vi "sonarPY.vi"(8 "error in (no error)":errorcluster, 11 "目標":dbl) -> (0 "error out":errorcluster, 3 "公分":dbl(slide) scale=0.0..200.0)   [LabVIEW 2019]
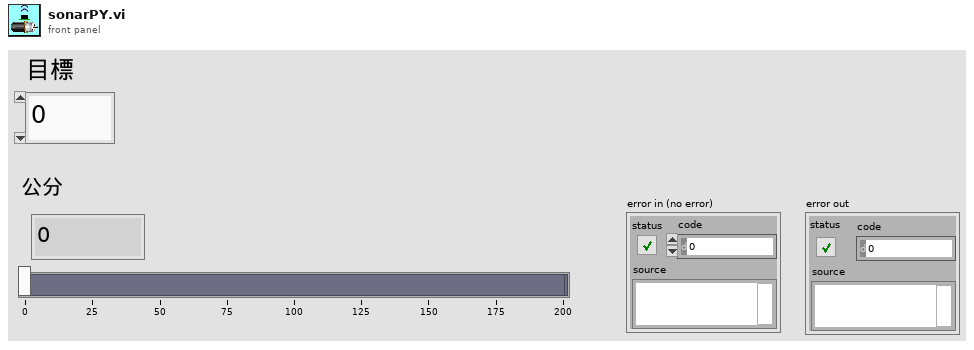
[diagram p1: front panel]
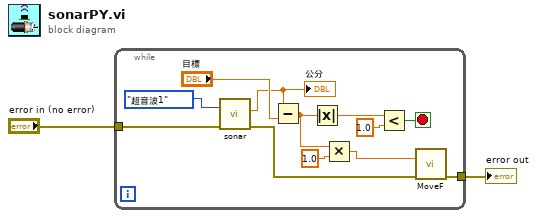
[diagram p0: block diagram]
diagram:
  n1 = while {
    tunnel: "error in (no error)" -> [w13]
    tunnel: [w7] -> w1
    stop <- w8 stop-if-true
    n2 = call "sonar.vi"("error in (no error)"=w13, "選擇超音波"=enum16{"請選擇超音波", "超音波1", "超音波2", "超音波3", "超音波4"}."超音波1") -> ("error out"=w6:errorcluster, "公分"=w5:dbl)  [unwired: 8 in]
    "公分" <- w5
    n3 = Subtract(x=w5, y="目標") -> (x-y=w11:dbl)
    n4 = Absolute Value(x=w11) -> (abs(x)=w10:dbl)
    n5 = Multiply(x=w11, y=1.0) -> (x*y=w3:dbl)
    n6 = Less?(x=w10, y=1.0) -> (x < y?=w8:bool)
    n7 = call "MoveF.vi"("Y"=w3, "error in (no error)"=w6) -> ("error out"=w7:errorcluster)  [unwired: 13 in]
  }
  "error out" <- w1
